vi "Page_Info_Validate_Filename.vi"(7 "message":string, 8 "error in (no error)":errorcluster, 9 "hasInvalidCharacters":bool, 10 "Filename":string, 11 "Build in":refnum<class "AB_Build.lvclass">) -> (0 "error out":errorcluster, 1 "hasInvalidCharacters":bool, 3 "Build out":refnum<class "AB_Build.lvclass">, 5 "message":string)   [LabVIEW 2020, in "AB_Deployment.lvlib"]
uses:
  <vilib>/AppBuilder/AB_Classes/Deployment/AB_Deployment.lvlib
  <vilib>/AppBuilder/AB_Classes/Build/AB_Build.lvclass
  <resource>/Framework/Providers/Common/provcom_StringGlobals.vi
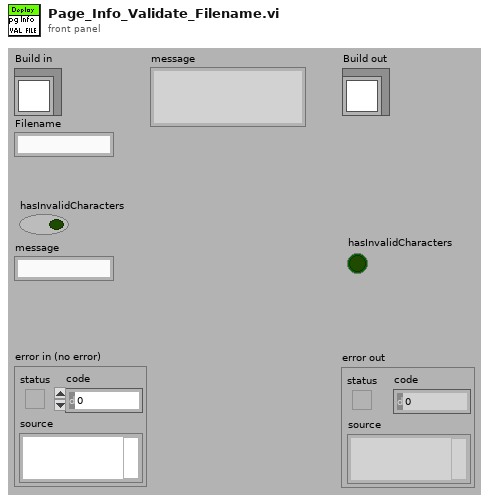
[diagram p1: front panel]
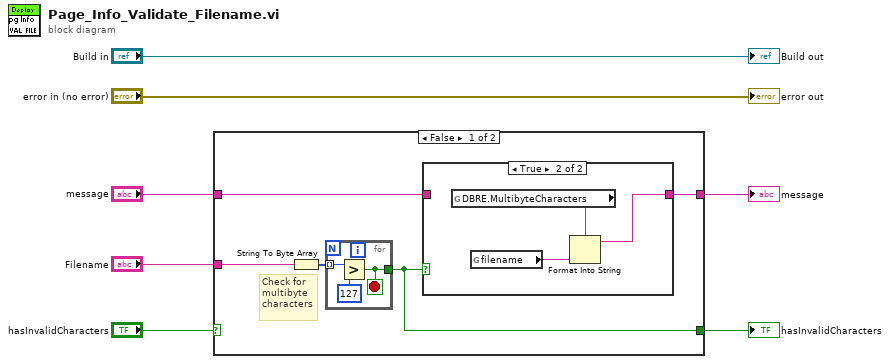
[diagram p0: block diagram]
diagram:
  n1 = case shown="False" "hasInvalidCharacters" {
    selector: "hasInvalidCharacters" -> [_ w21]
    tunnel: "Filename" -> [w11 _]
    tunnel: [w10 w21] -> w4
    tunnel: [w9 w20] -> w5
    tunnel: "message" -> [w8 w20]
    frame False {
      # "Check for\nmultibyte\ncharacters"
      n2 = String To Byte Array(string=w11) -> (unsigned byte array=w12:u8[])
      n3 = for {
        tunnel: w12 -> [w19] mode=indexing
        tunnel: [w17] -> w10
        stop <- w17 stop-if-true
        n4 = Greater?(x=w19, y=u8 127) -> (0:w17:bool)
      }
      n5 = case shown="True" w10 {
        tunnel: [w13 w15] -> w9
        tunnel: w8 -> [w13 _]
        frame False {
        }
        frame True {
          n6 = global read "provcom_StringGlobals.vi" "DBRE.MultibyteCharacters"() -> (w14:string)
          n7 = global read "provcom_StringGlobals.vi" "filename"() -> (w16:string)
          n8 = Format Into String(format string=w14, w16) -> (resulting string=w15:string)  [unwired: 2 in, 1 out]
        }
      }
    }
    frame True {
    }
  }
  "message" <- w5
  "hasInvalidCharacters" <- w4
  "error out" <- "error in (no error)"
  "Build out" <- "Build in"
